vi "error_check_shutdown_temp_cont.vi"(8 "f":T1, 11 "Boolean":bool) -> (3 "s? t:f":T1)   [LabVIEW 2017]
uses:
  controls/State.ctl
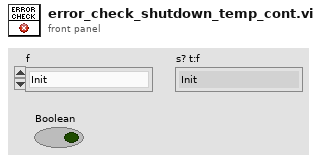
[diagram p1: front panel]
types:
  T1 = typedef "State.ctl" = enum16{"Init", "Idle", "Shutdown"}
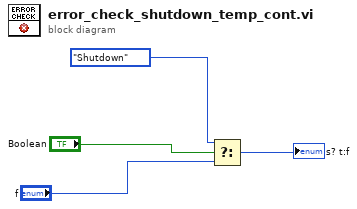
[diagram p0: block diagram]
diagram:
  n1 = Select(t=State."Shutdown" ("States"), s="Boolean", f="f") -> (s? t:f=→"s? t:f":T1)
